vi "Signal Generator_5761.vi"(0 "Register":refnum<k21>="PatternGenerator", 1 "FPGA I/O In":refnum<k21>="IO Module\\DDCA_Port2_Write", 2 "Drive?":bool, 3 "Enabled":bool, 4 "Clock in":refnum<k21>="100 MHz Clock", 5 "SGNumber":i16) -> ()   [LabVIEW 2013, in "IRIO.lvlib"]
uses:
  IRIO.lvlib
  <vilib>/Platform/TimedLoop/XDataNode/timing_clust.ctl
  <vilib>/Platform/TimedLoop/XDataNode/nitl_modes.ctl
  <vilib>/Platform/TimedLoop/XDataNode/wakeup.ctl
  <vilib>/rvi/Emulation/niFpgaSctlEmulationGetInTimedLoop.vi
  <vilib>/rvi/Emulation/niFpgaEmulationReportErrorSimple.vi
  <vilib>/rvi/Emulation/niFpgaGetClockAttributes.vi
  <vilib>/rvi/Emulation/niFpgaCriticalErrorInLSC.vi
  <vilib>/rvi/DataTransferAndStorage/Container/Common/niFpgaContainerExecOnDevCompGetState.vi
  <vilib>/rvi/DataTransferAndStorage/Register/Emulation/niFpgaRegisterEmulationFpgaImpl.vi
  <instcachedir>/0/niFpgaRegisterEmulationFpgaImpl_DCF4BC0110594B98B44A971D60CEEC4D.lvgen/niFpgaRegisterEmulationFpgaImpl_DCF4BC0110594B98B44A971D60CEEC4D_008.vi
  <vilib>/rvi/DataTransferAndStorage/Container/Common/niFpgaContainerGetUniqueNameForEmu.vi
  <vilib>/rvi/Emulation/niFpgaProcessEmulError.vi
  <vilib>/rvi/eio/common/nirviEmuTemplateMethod_errors.vi
  <vilib>/Platform/TimedLoop/XDataNode/XDataNode.xnode
  <vilib>/rvi/DataTransferAndStorage/Container/XNode/niFpgaContainer.xnode
  <vilib>/rvi/DataTransferAndStorage/Register/Emulation/niFpgaRegisterEmulationRefIn.vi
  <vilib>/eio/EIONode/EIONode.xnode
  <vilib>/Platform/TimedLoop/XDataNode/XDNodeRunTimeDep.lvlib
  common/GlobalReg.vi
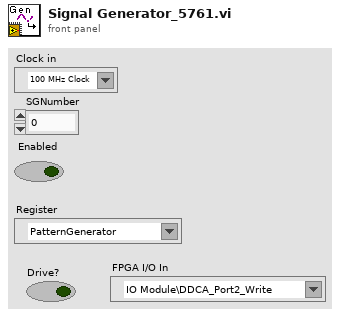
[diagram p1: front panel]
types:
  T1 = typedef "XDNodeRunTimeDep.lvlib/timing_clust.ctl" = cluster{"Expected End [f-1]":u64, "Actual End [f-1]":u64, "Finished Late? [f-1]":bool, "Expected End [i-1]":u64, "Actual End [i-1]":u64, "Finished Late? [i-1]":bool, "Expected Start [i]":u64, "Actual Start [i]":u64, "Expected Start [f]":u64, "Actual Start [f]":u64, "Source Name":string, "Structure Name":string, "Period":i64, "Deadline":i64, "Offset":i64, "Start":i64, "Priority":i32, "Timeout":i32, "Mode":T2, "Wakeup Reason":T3, "Error":errorcluster, "Source Type":string, "Secondary Source Type":string, "Global End Time":u64, "Global Start Time":u64, "Frame Duration":u64, "Iteration Duration":u64, "Assigned CPU":i32, "I/O Scan Engine Mode":u32}
  T2 = typedef "XDNodeRunTimeDep.lvlib/nitl_modes.ctl" = enum32{"No Change", "Process missed periods, maintain original phase", "Discard missed periods, maintain original phase", "Process missed periods, ignore original phase", "Discard missed periods, ignore original phase"}
  T3 = typedef "XDNodeRunTimeDep.lvlib/wakeup.ctl" = enum32{"Normal", "Aborted", "Asynchronous wakeup", "Timing source error", "Timed loop error", "Timeout"}
  T4 = cluster{"AOEnable":bool, "AO0":i32, "SGUpdateRate":u32, "SGPhase":u32, "SGFreq":u32, "SGAmp":u16, "SGSignalType":u8, "N":u8}
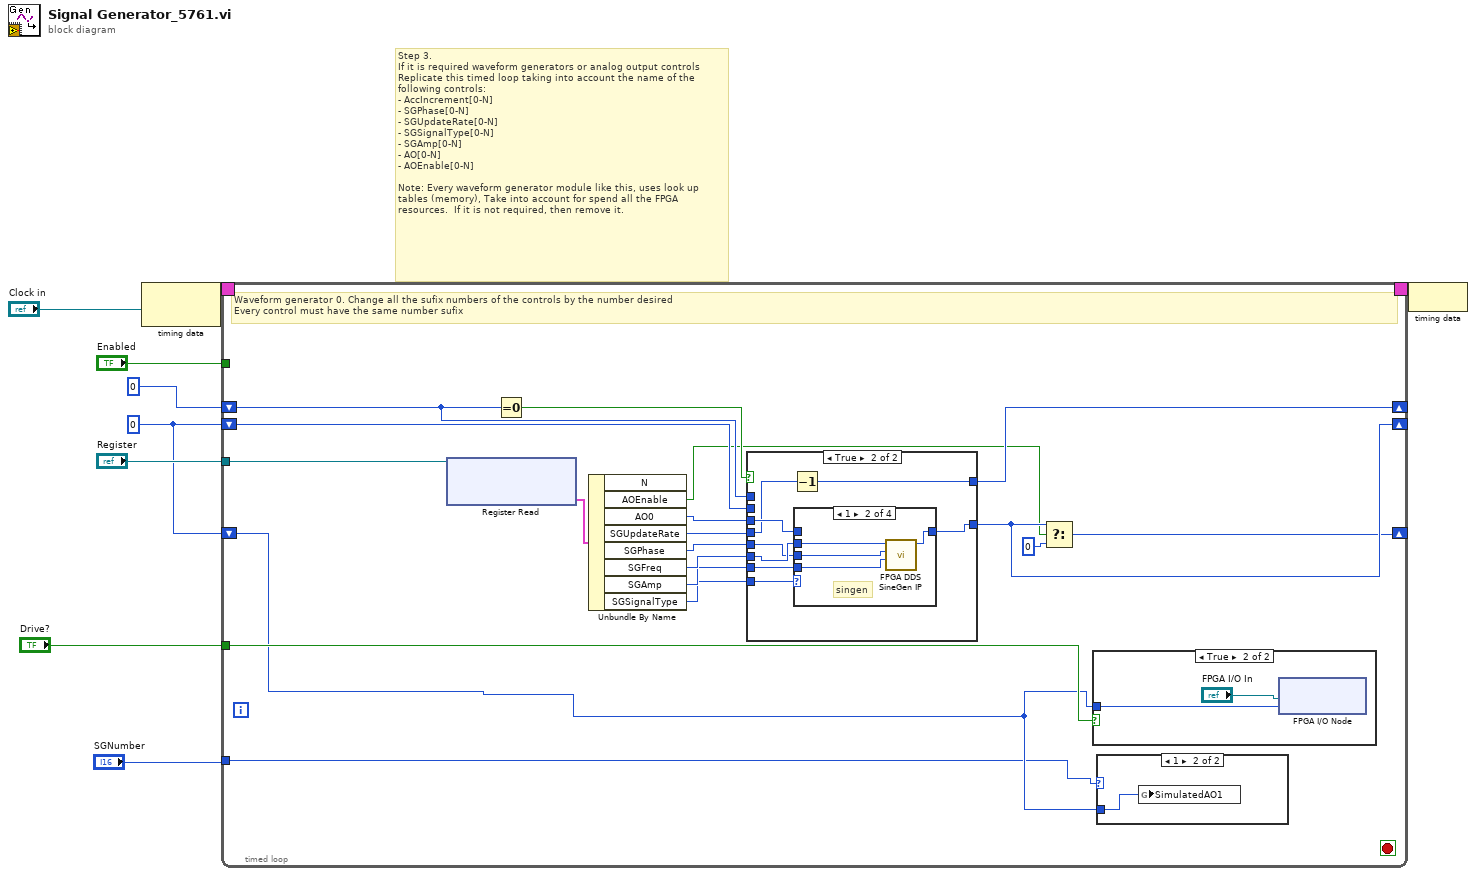
[diagram p0: block diagram]
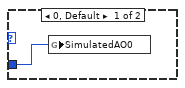
[diagram p2: hidden frame]
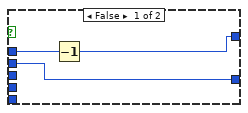
[diagram p4: hidden frame]
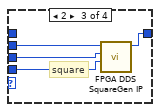
[diagram p6: hidden frame]
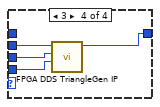
[diagram p7: hidden frame]
diagram:
  w2 = 0 ("Signal Value")
  # "Step 3.\nIf it is required waveform generators or analog output controls\nReplicate this timed loop taking into account the name of the \nfollowing controls:\n- AccIncrement[0-N]\n- SGPhase[0-N]\n- SGUpdateRate[0-N]\n- SGSignalType[0-N]\n- SGAmp[0-N]\n- AO[0-N]\n- AOEnable[0-N]\n\nNote: Every waveform generator module like this, uses look up tables (memory), Take into account for spend all the FPGA resources.  If it is not required, then remove it."
  n1 = node-c288("Clock in") -> (w9:T1)
  n2 = timed-loop {
    shift-right: [w18] -> _
    shift-left: w2 -> [w20]
    timing: w9 -> [_]
    timing-out: [_] -> w8
    shift-right: [w28] -> _
    shift-left: u32 0 -> [w19]
    tunnel: "Enabled" -> [_]
    tunnel: "Drive?" -> [w17]
    tunnel: "Register" -> [w13]
    shift-right: [w12] -> _
    shift-left: w2 -> [w11]
    tunnel: "SGNumber" -> [w10]
    stop <- _ stop-if-true
    # "Waveform generator 0. Change all the sufix numbers of the controls by the number desired\nEvery control must have the same number sufix"
    n3 = xnode ("Register Read")("Register In"=w13) -> ("Data"=w14:T4)  [unwired: 1 out]
    n4 = Equal To 0?(x=w19) -> (x = 0?=w21:bool)
    n5 = Unbundle By Name(w14) -> ("AOEnable"=w15:bool, "AO0"=w22:i32, "SGUpdateRate"=w23:u32, "SGPhase"=w26:u32, "SGFreq"=w27:u32, "SGAmp"=w25:u16, "SGSignalType"=w24:u8)  [unwired: 1 out]
    n6 = case shown="True" w21 {
      tunnel: w27 -> [_ w43]
      tunnel: w26 -> [_ w42]
      tunnel: w25 -> [_ w41]
      tunnel: [w35 w40] -> w18
      tunnel: w19 -> [w34 _]
      tunnel: [w33 w36] -> w28
      tunnel: w20 -> [w35 _]
      tunnel: w24 -> [_ w39]
      tunnel: w23 -> [_ w37]
      tunnel: w22 -> [_ w38]
      frame False {
        n7 = Decrement(x=w34) -> (x-1=w33:u32)
      }
      frame True {
        n8 = Decrement(x=w37) -> (x-1=w36:u32)
        n9 = case shown="1" w39 {
          tunnel: w43 -> [_ w48 w52 w56]
          tunnel: w42 -> [_ w47 w51 w55]
          tunnel: w41 -> [_ w46 w50 w54]
          tunnel: [w44 w45 w49 w53] -> w40
          tunnel: w38 -> [w44 _ _ _]
          frame 0, Default {
          }
          frame 1 {
            # "singen"
            n10 = call "FPGA DDS SineGen IP.vi"("Signal Amplitude (x 2^15)"=w46, "Phase Shift"=w47, "Accumulator Increment"=w48) -> ("Signal Value"=w45:i16)  [unwired: 7 in, 1 out]
          }
          frame 2 {
            # "square"
            n11 = call "FPGA DDS SquareGen IP.vi"("Signal Amplitude (x 2^15)"=w50, "Phase Shift"=w51, "Accumulator Increment"=w52) -> ("Signal Value"=w49:i16)  [unwired: 7 in, 1 out]
          }
          frame 3 {
            n12 = call "FPGA DDS TriangleGen IP.vi"("Signal Amplitude (x 2^15)"=w54, "Phase Shift"=w55, "Accumulator Increment"=w56) -> ("Signal Value"=w53:i16)  [unwired: 7 in, 1 out]
          }
        }
      }
    }
    n13 = Select(t=w18, s=w15, f=0) -> (s? t:f=w12:i32)
    n14 = case shown="True" w17 {
      tunnel: w11 -> [_ w32]
      frame False {
      }
      frame True {
        n15 = xnode "FPGA I/O Node"("I/O Item"=w32, "FPGA I/O In"="FPGA I/O In") -> ()  [unwired: 1 out]
      }
    }
    n16 = case shown="1" w10 {
      tunnel: w11 -> [w29 w30]
      frame 0, Default {
        n17 = global write "GlobalReg.vi" "SimulatedAO0"(w29) -> ()
      }
      frame 1 {
        n18 = global write "GlobalReg.vi" "SimulatedAO1"(w30) -> ()
      }
    }
  }
  n19 = node-c288(w8) -> ()
